vi "fgv_stop-point_temp-buffer.vi"(7 "cmd":enum16{"init", "upload", "read", "del"}(ring), 10 "arrive point":cluster{dbl, dbl}, 11 "stop pt array":cluster{dbl, dbl}[](array[cluster])) -> (3 "stop pt update out":cluster{dbl, dbl}[](array[cluster]) {"?" format="%.13f"; "?" format="%.13f"})   [LabVIEW 2019]
panel:
  out "stop pt in":cluster{dbl, dbl}[](array[cluster]) {"?" format="%.13f"; "?" format="%.13f"}
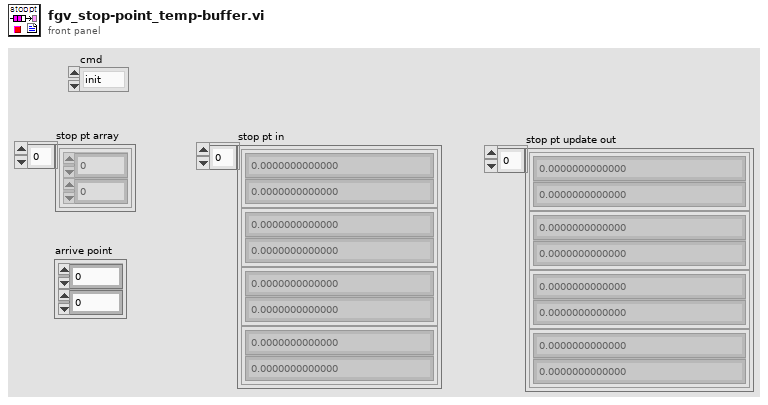
[diagram p1: front panel]
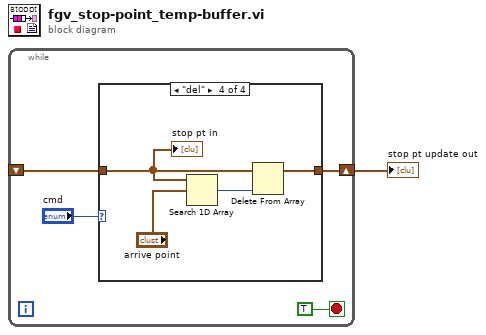
[diagram p0: block diagram]
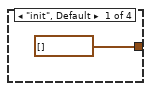
[diagram p2: hidden frame]
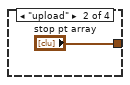
[diagram p3: hidden frame]
diagram:
  n1 = while {
    shift-right: [w3] -> w1
    shift-left: _ -> [w2]
    stop <- TRUE stop-if-true
    n2 = case shown="\"del\"" "cmd" {
      tunnel: [cluster{dbl, dbl}[] [] ("stop pt array") "stop pt array" w8 w12] -> w3
      tunnel: w2 -> [_ _ w8 w9]
      frame "init", Default {
      }
      frame "upload" {
      }
      frame "read" {
      }
      frame "del" {
        n3 = Search 1D Array(1D array=w9, element="arrive point") -> (index of element=w10:i32)  [unwired: 1 in]
        n4 = Delete From Array(array=w9, index=w10) -> (array with subset deleted=w12:cluster{dbl, dbl}[])  [unwired: 1 in, 1 out]
        "stop pt in" <- w9
      }
    }
  }
  "stop pt update out" <- w1
